vi "OAT Order Magnitude and Phase (Even Angle Signal, 1 Channel).vi"(0 "even-angle signal":cluster{"r0":dbl, "dr":dbl, "Y":dbl[]}={"r0"=0.0, "dr"=1.0, "Y"=[]} {"r0" format="%.2p"; "dr" format="%.2p"; "Y" format="%.2f"}, 1 "x-axis selection":u16(ring)=2 items=["Time", "Revolution", "RPM"], 2 "reset? (F)":bool, 5 "even-angle channel info":T8={"channel name"="", "description"="", " channel info"={"sensor sensitivity"=1000.0, "engineering units"=1, "dB reference"=1.0, "custom label"="EU", "weighting filter"=0, "pregain"=0.0}} {"channel info"."pregain" format="%.2f"; "channel info"."weighting filter" items=["Linear", "A-weighting", "B-weighting", "C-weighting", "ITU-R 468-4", "Dolby", "CCITT", "C-message", "Wb", "Wc", "Wd", "We", "Wf", "Wh", "Wj", "Wk", "Wm", "AES17 20 kHz lowpass", "AES17 40 kHz lowpass", "AES17 20 kHz highpass", "AES17 40 kHz highpass"]; "channel info"."dB reference" format="%^.1e"; "channel info"."engineering units" items=["custom..."=0, "V"=1, "A"=21, "C"=30, "pC"=31, "s"=32, "-"=29, "Pa"=2, "N"=20, "g"=3, "m/s^2"=4, "m/s"=5, "m"=6, "mm/s"=12, "mm"=13, "micron/s"=14, "micron"=15, "in/s^2"=7, "in/s"=8, "in"=9, "mil/s"=10, "mil"=11, "rad/s^2"=16, "rad/s"=17, "rad"=18, "deg/s^2"=26, "deg/s"=27, "deg"=28, "RPM"=22, "cycle/s^2"=23, "Hz"=24, "cycle"=25, "strain"=19]; "channel info"."sensor sensitivity" format="%#_5f"}, 7 "even-angle position info":T1, 9 "orders to compute (1.0)":dbl[](array[numeric])=[1.0] format="%.2f", 11 "error in (no error)":errorcluster, 12 "bandwidth [order]":dbl=1.0 format="%.2f", 13 "view":T12={"dB on? (F)"=FALSE, "unwrap phase? (T)"=TRUE, "unit in degree? (T)"=TRUE}, 14 "zero delay? (F)":bool) -> (3 "unit labels":T10, 4 "magnitudes [RMS]":T11(array[cluster]) {"magnitude" format="%.2f"; "time/rev/rpm" format="%.2f"}, 6 "phases [phase lag]":cluster{"time/rev/rpm":dbl[], "phase":dbl[]}[](array[cluster]) {"phase" format="%.2f"; "time/rev/rpm" format="%.2f"}, 8 "magnitude/phase position info":T1, 10 "magnitude info":T2={"channel name"="", "description"="", "x-axis units"=0, "spectral info"={"spectrum type"=enum."Power [Magnitude^2]", "linear/dB"=enum."linear", "window"=0, "window size"=0, "FFT size"=0}, "engineering units"=1, "custom label"="", "dB reference [EU]"=0.0, "peak units"=enum."rms", "weighting filter"=0, "spectral density?"=FALSE, "unit label"="", "spectrum skewed?"=FALSE, "complimentary spectrum units"=enum."none"} {"x-axis units" items=["Time (s)"=0, "Frequency-CB (Hz)"=1, "Frequency-CPB (Hz)"=1248, "Frequency-Arbitrary (Hz)"=2357, "Quefrency (s)"=2, "Revolutions (rev)"=3, "Order"=4, "Speed (RPM)"=11, "Speed (rad/s)"=21, "Index"=65535]; "weighting filter" items=["Linear", "A-weighting", "B-weighting", "C-weighting", "ITU-R 468-4", "Dolby", "CCITT", "C-message", "Wb", "Wc", "Wd", "We", "Wf", "Wh", "Wj", "Wk", "Wm", "AES17 20 kHz lowpass", "AES17 40 kHz lowpass", "AES17 20 kHz highpass", "AES17 40 kHz highpass"]; "dB reference [EU]" format="%.2f"; "engineering units" items=["custom..."=0, "V"=1, "A"=21, "C"=30, "pC"=31, "s"=32, "-"=29, "Pa"=2, "N"=20, "g"=3, "m/s^2"=4, "m/s"=5, "m"=6, "mm/s"=12, "mm"=13, "micron/s"=14, "micron"=15, "in/s^2"=7, "in/s"=8, "in"=9, "mil/s"=10, "mil"=11, "rad/s^2"=16, "rad/s"=17, "rad"=18, "deg/s^2"=26, "deg/s"=27, "deg"=28, "RPM"=22, "cycle/s^2"=23, "Hz"=24, "cycle"=25, "strain"=19]; "spectral info"."window" items=["None "=0, "Hanning"=1, "Hamming"=2, "Blackman-Harris"=3, "Exact Blackman"=4, "Blackman"=5, "Flat Top"=6, "4 Term B-Harris "=7, "7 Term B-Harris"=8, "Low Sidelobe"=9, "Force - Exponential"=10, "Gaussian"=62]}, 15 "error out":errorcluster)   [LabVIEW 2017, in "SoundVib_OrderTracking.lvlib"]
doc: "Computes the magnitudes and phases of designated orders in an even-angle signal. Use this VI to track particular orders specified by <B>orders to compute</B>. Wire data to the <B>even-angle signal</B> input to determine the polymorphic instance to use or manually select the instance."
uses:
  <vilib>/addons/Sound and Vibration/Order Analysis/Resample Order Tracking/SoundVib_OrderTracking.lvlib
  <vilib>/addons/Sound and Vibration/Order Analysis/Misc/OAT Position Info.ctl
  <vilib>/addons/_NISVFA/_Shared subVIs/Controls/svc_Resampled Channel Info.ctl
  <vilib>/addons/_NISVFA/_Shared subVIs/Controls/svc_Channel Info.ctl
  <vilib>/addons/_NISVFA/_Shared subVIs/Controls/svc_Engineering Units Text Ring.ctl
  <vilib>/addons/_NISVFA/_Shared subVIs/Controls/svc_Weighting Filter Text Ring.ctl
  <vilib>/addons/_NISVFA/_Shared subVIs/Controls/svc_Spectrum Info.ctl
  <vilib>/addons/_NISVFA/_Shared subVIs/Controls/svc_X-Axis Units.ctl
  <vilib>/addons/_NISVFA/_Shared subVIs/Controls/svc_Spectrum Type.ctl
  <vilib>/addons/_NISVFA/_Shared subVIs/Controls/svc_Complimentary Spectrum Units.ctl
  <vilib>/addons/Sound and Vibration/Order Analysis/Resample Order Tracking/SubVIs/OAT Order Magnitude and Phase Plot(XY) (Single Channel).vi
  <vilib>/addons/Sound and Vibration/Order Analysis/Resample Order Tracking/SubVIs/OAT Demodulate Multiple Orders (Single Channel).vi
  <vilib>/addons/Sound and Vibration/Order Analysis/Resample Order Tracking/SubVIs/OAT Verify Resampled Signal (OMP, Single Channel).vi
  <vilib>/addons/Sound and Vibration/Order Analysis/Resample Order Tracking/SoundVib_Resampling.lvlib
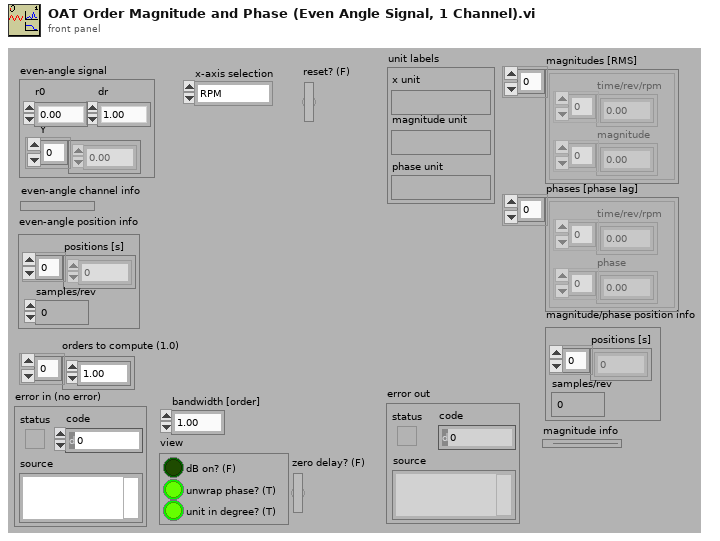
[diagram p1: front panel]
types:
  T1 = typedef "OAT Position Info.ctl" = cluster{"positions [s]":dbl[], "samples/rev":dbl}
  T2 = typedef "svc_Spectrum Info.ctl" = cluster{"channel name":string, "description":string, "x-axis units":T3, "spectral info":cluster{"spectrum type":T4, "linear/dB":enum16{"linear", "dB"}, "window":u16, "window size":i32, "FFT size":i32}, "engineering units":T5, "custom label":string, "dB reference [EU]":dbl, "peak units":enum16{"rms", "peak", "peak-peak"}, "weighting filter":T6, "spectral density?":bool, "unit label":string, "spectrum skewed?":bool, "complimentary spectrum units":T7}
  T3 = typedef "svc_X-Axis Units.ctl" = u16
  T4 = typedef "svc_Spectrum Type.ctl" = enum16{"FFT Spectrum [complex]", "Amplitude [Magnitude]", "Power [Magnitude^2]", "Cross Spectrum [complex]", "Frequency Response [Complex]"}
  T5 = typedef "svc_Engineering Units Text Ring.ctl" = u16
  T6 = typedef "svc_Weighting Filter Text Ring.ctl" = u16
  T7 = typedef "svc_Complimentary Spectrum Units.ctl" = enum16{"none", "radians", "degrees", "cycles", "imaginary"}
  T8 = typedef "svc_Resampled Channel Info.ctl" = cluster{"channel name":string, "description":string, " channel info":T9}
  T9 = typedef "svc_Channel Info.ctl" = cluster{"sensor sensitivity":dbl, "engineering units":T5, "dB reference":dbl, "custom label":string, "weighting filter":T6, "pregain":dbl}
  T10 = cluster{"x unit":string, "magnitude unit":string, "phase unit":string}
  T11 = cluster{"time/rev/rpm":dbl[], "magnitude":dbl[]}[]
  T12 = cluster{"dB on? (F)":bool, "unwrap phase? (T)":bool, "unit in degree? (T)":bool}
  T13 = cluster{"X unit":string, "unit label":string, "unit label":string}
  T14 = cluster{"unwrap phase? (T)":bool, "unit in degree? (T)":bool}
  T15 = cluster{"bandwidth [order] out":dbl, "stop band attenuation":u16}
  T16 = typedef "SoundVib_TachProcess.lvlib/speed profile.ctl" = cluster{"time [s]":dbl[], "speed [RPM]":dbl[]}
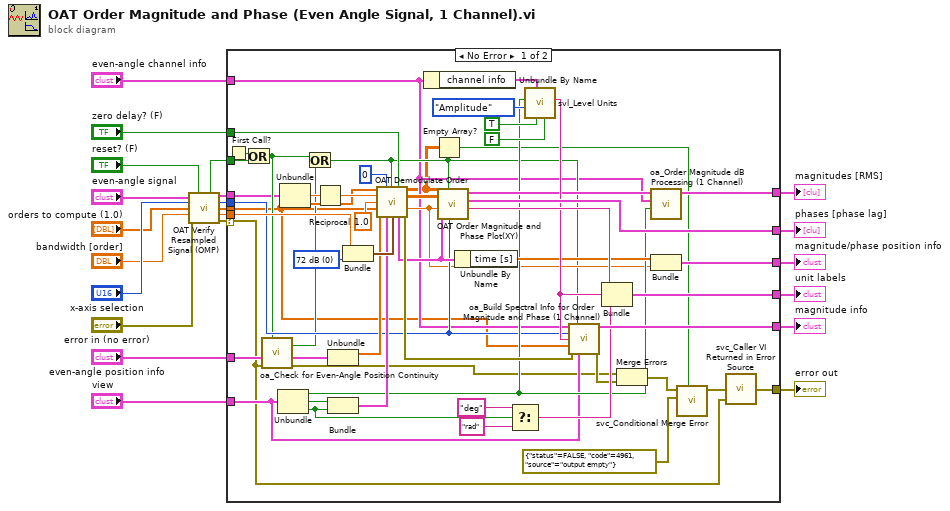
[diagram p0: block diagram]
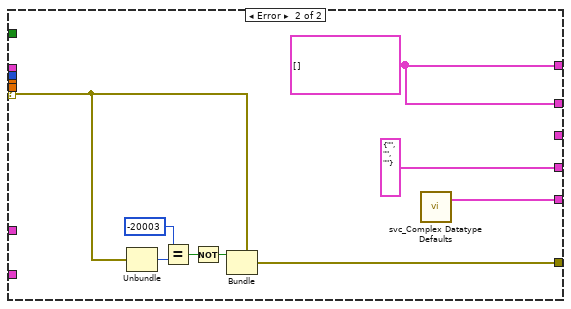
[diagram p2: hidden frame]
diagram:
  n1 = call-poly <vilib>:"OAT Verify Resampled Signal (OMP).vi"("resampled signal"="even-angle signal", "reset in (T)"="reset? (F)", "X axis selection"="x-axis selection", "orders to compute (1.0)"="orders to compute (1.0)", "bandwidth [order]"="bandwidth [order]", "error in (no error)"="error in (no error)") -> ("reset out (T)"=w11:bool, "resampled signal dup"=w13:cluster{"r0":dbl, "dr":dbl, "Y":dbl[]}, "X axis selection out"=w2:u16, "orders to compute (1.0) out"=w4:dbl[], "bandwidth [order] out"=w3:dbl, "error out"=w10:errorcluster)  [unwired: 4 in]
  n2 = case shown="No Error" w10 {
    selector: w10 -> [w23 w80]
    tunnel: [w77 T13 {"X unit"="", "unit label"="", "unit label"=""}] -> w22
    tunnel: "even-angle position info" -> [w32 _]
    tunnel: "view" -> [w42 _]
    tunnel: [w76 w86] -> w19
    tunnel: [w52 w86] -> w18
    tunnel: w13 -> [w33 _]
    tunnel: [w24 w79] -> w17
    tunnel: [w75 w78] -> w16
    tunnel: [w74 _] -> w15
    tunnel: w11 -> [w50 _]
    tunnel: "even-angle channel info" -> [w34 _]
    tunnel: w4 -> [w30 _]
    tunnel: w3 -> [w44 _]
    tunnel: w2 -> [w43 _]
    tunnel: "zero delay? (F)" -> [w39 _]
    frame No Error {
      w59 = u16 0 items=["72 dB", "96 dB", "120 dB"] ("stop band attenuation")
      n3 = First Call?() -> (First Call?: T/F=w49:bool)
      n4 = Or(x=w49, y=w50) -> (x .or. y?=w37:bool)
      n5 = call <vilib>:"oa_Check for Even-Angle Position Continuity.vi"("reset in"=w37, "error in (no error)"=w23, "even-angle position info"=w32) -> ("error out"=w38:errorcluster, "even-angle position info dup"=w31:T1, "position not continuous"=w36:bool)  [unwired: 6 in]
      n6 = Unbundle(w42) -> ("dB on? (F)"=w45:bool, "unwrap phase? (T)"=w51:bool, "unit in degree? (T)"=w48:bool)
      n7 = Unbundle(w33) -> ("dr"=w73:dbl, "Y"=w65:dbl[])  [unwired: 1 out]
      n8 = Or(x=w37, y=w36) -> (x .or. y?=w35:bool)
      n9 = Reciprocal(x=w73) -> (1/x=w66:dbl)
      n10 = Unbundle(w31) -> ("positions [s]"=w56:dbl[])  [unwired: 1 out]
      n11 = Bundle("unwrap phase? (T)"=w51, "unit in degree? (T)"=w48) -> (w54:T14)  [unwired: 1 in]
      n12 = Bundle("bandwidth [order] out"=w44, "stop band attenuation"=w59) -> (w58:T15)  [unwired: 1 in]
      n13 = call-poly <vilib>:"OAT Demodulate Order.vi"("Y"=w65, "decimation factor"=0 ("decimation factor (auto)"), "reset? (True)"=w35, "zero delay? (F)"=w39, "samples/rev"=w66, "samples/rev wanted"=1.0 ("x"), "orders (1.0)"=w30, "time stamps in"=w56, "phase setting"=w54, "order info"=w58) -> ("magnitudes (RMS)"=w29:dbl[][], "phase lag"=w67:dbl[][], "samples/rev"=w41:dbl, "speed profile"=w57:T16, "error out"=w61:errorcluster)  [unwired: 1 in]
      n14 = Unbundle By Name(w34) -> ("channel info"=w62:T9)
      n15 = Empty Array?(array=w29) -> (empty?=w27:bool)
      n16 = call-poly <vilib>:"OAT Order Magnitude and Phase Plot(XY).vi"("X axis selection"=w43, "reset? (True)"=w35, "speed profile"=w57, "samples/rev"=w41, "phase lag  (even angular)"=w67, "magnitudes (even angular)"=w29) -> ("X unit"=w72:string, "phase lag"=w76:cluster{"X":dbl[], "Y":dbl[]}[], "magnitudes"=w53:cluster{"X":dbl[], "Y":dbl[]}[])  [unwired: 3 in]
      n17 = Unbundle By Name(w57) -> ("time [s]"=w55:dbl[])
      n18 = Select(t="deg" ("unit label"), s=w48, f="rad" ("unit label")) -> (s? t:f=w68:string)
      n19 = call <vilib>:"svl_Level Units.vi"("include weighting if dB On FALSE"=FALSE, "rms level (T)"=TRUE, "channel info"=w62, "view mode"=enum16{"Power", "Amplitude"}."Amplitude", "dB On (T)"=w45) -> ("unit label"=w60:string)  [unwired: 4 in, 2 out]
      n20 = call <vilib>:"oa_Build Spectral Info for Order Magnitude and Phase (1 Channel).vi"("resampled channel info"=w34, "reset? (T)"=w35, "X axis selection"=w43, "unit label"=w60, "orders to compute"=w30, "error in (no error)"=w61, "view"=w42) -> ("spectrum info"=w75:T2, "error out"=w40:errorcluster)  [unwired: 7 in]
      n21 = Bundle("X unit"=w72, "unit label"=w60, "unit label"=w68) -> (w77:T13)  [unwired: 1 in]
      n22 = Merge Errors(w38, w40) -> (w26:errorcluster)
      n23 = call <vilib>:"oa_Order Magnitude dB Processing (1 Channel).vi"("dB on? (T)"=w45, "even angle channel info"=w34, "magnitudes"=w53) -> ("magnitudes dB"=w52:T11)  [unwired: 8 in]
      n24 = Bundle("time [s]"=w55, "samples/rev"=w41) -> (w74:cluster{"time [s]":dbl[], "samples/rev":dbl})  [unwired: 1 in]
      n25 = call <vilib>:"svc_Conditional Merge Error.vi"("merge"=w27, "new error"=errorcluster {"status"=FALSE, "code"=4961, "source"="output empty"}, "error in (no error)"=w26) -> ("error out"=w25:errorcluster)  [unwired: 8 in]
      n26 = call <vilib>:"svc_Caller VI Returned in Error Source.vi"("warning input to caller"=w23, "error in (no error)"=w25) -> ("error out"=w24:errorcluster)  [unwired: 3 in]
    }
    frame Error {
      w86 = cluster{"X":dbl[], "Y":dbl[]}[] [] ("magnitudes")
      n27 = Unbundle(w80) -> ("code"=w84:i32)  [unwired: 2 out]
      n28 = Equal?(x=-20003 ("t"), y=w84) -> (x = y?=w82:bool)
      n29 = Not(x=w82) -> (.not. x?=w81:bool)
      n30 = Bundle(cluster=w80, "status"=w81) -> (w79:errorcluster)  [unwired: 2 in]
      n31 = call <vilib>:"svc_Complex Datatype Defaults.vi"() -> ("dead spectrum info"=w78:T2)  [unwired: 11 in, 8 out]
    }
  }
  "magnitudes [RMS]" <- w18
  "phases [phase lag]" <- w19
  "unit labels" <- w22
  "error out" <- w17
  "magnitude info" <- w16
  "magnitude/phase position info" <- w15
